vi "test_datasocket.vi"() -> ()   [LabVIEW 2023]
uses:
  <vilib>/ActorFramework/Actor/Actor.lvclass
  AI/AI Simulated CFGs/AI DAQmx Cont CFG Simulated.lvclass
  <vilib>/ni/Actors/Network Endpoint Actors/Protocols/Network Stream Strategy/Netowrk Stream Listener/Network Stream Listener.lvclass
  MSS Target/MSS Target Actor/MSS Target Actor.lvclass
  AI/AI Cont CFG/AI DAQmx Cont CFG.lvclass
  C:/Program Files/National Instruments/LabVIEW 2023/vi.lib/ni/Actors/Network Endpoint Actors/Protocols/Network Stream Strategy/Network Stream/Network Stream.lvclass
  C:/Program Files/National Instruments/LabVIEW 2023/vi.lib/ni/Actors/Network Endpoint Actors/Abstract Classes/Message Stream/Message Stream.lvclass
  C:/Program Files/National Instruments/LabVIEW 2023/vi.lib/ni/Actors/Network Endpoint Actors/Protocols/Network Stream Strategy/Netowrk Stream Listener/Network Stream Listener.lvclass
  C:/Program Files/National Instruments/LabVIEW 2023/vi.lib/ActorFramework/Actor/Actor.lvclass
  D:/git/HAL/HAL GOOP4/MSS Target/MSS Target Actor/MSS Target Actor.lvclass
  D:/git/HAL/HAL GOOP4/MSS Target/IMSS Target Actor/IMSS Target Actor.lvclass
  C:/Program Files/National Instruments/LabVIEW 2023/vi.lib/ni/Actors/Network Endpoint Actors/Nested Endpoint Caller/Nested Endpoint Caller/Nested Endpoint Caller.lvclass
panel:
  out "error out":errorcluster
  in  "error in":errorcluster
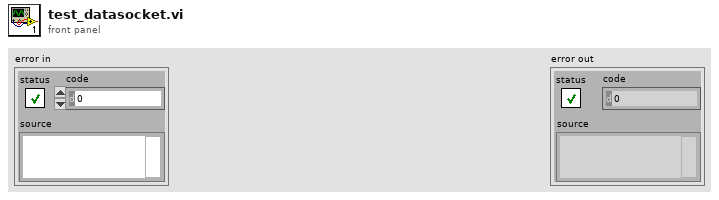
[diagram p1: front panel]
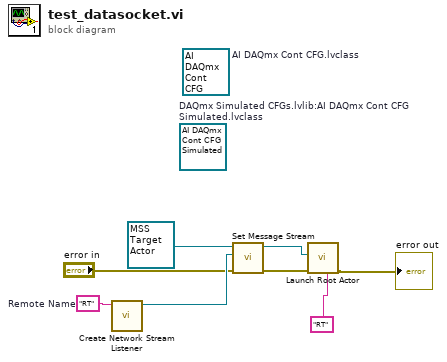
[diagram p0: block diagram]
diagram:
  (unwired) refnum<class "AI DAQmx Cont CFG.lvclass"> refnum  # AI DAQmx Cont CFG.lvclass
  w7 = "RT"  # Remote Name
  (unwired) refnum<class "AI DAQmx Cont CFG Simulated.lvclass"> refnum  # DAQmx Simulated CFGs.lvlib:AI DAQmx Cont CFG Simulated.lvclass
  n1 = call <vilib>:"Create Network Stream Listener.vi"("Name"=w7) -> ("Network Stream Listener"=w5:refnum<class "Network Stream Listener.lvclass">)  [unwired: 10 in]
  n2 = call "Set Message Stream.vi"("Message Stream.lvclass"=w5, "CRIO MSS Test Actor in"=refnum<class "MSS Target Actor.lvclass"> refnum ("MSS Target Actor.lvlib:MSS Target Actor.lvclass")) -> ("CRIO MSS Test Actor out"=w4:refnum<class "MSS Target Actor.lvclass">)  [unwired: 9 in]
  n3 = call <vilib>:"Launch Root Actor.vi"("Debug Alias"="RT", "error in (no error)"="error in", "Actor"=w4) -> ("error out"=→"error out":errorcluster)  [unwired: 7 in, 1 out]
